vi "AlazarGetBoardKind.vi"(0 "Handle":u64, 1 "error in (no error)":errorcluster) -> (2 "Handle":u64, 3 "Board Kind":u32, 4 "Return Code":u32, 5 "error out":errorcluster)   [LabVIEW 2009]
doc: "Get a board model identifier of the board associated with a board handle."
uses:
  ATSApi.dll
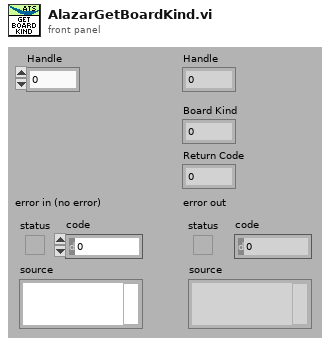
[diagram p1: front panel]
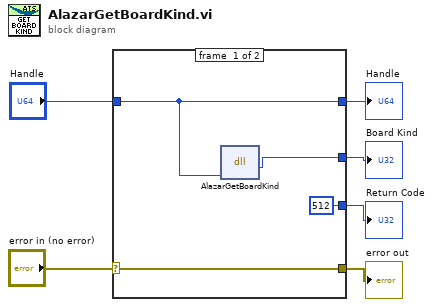
[diagram p0: block diagram]
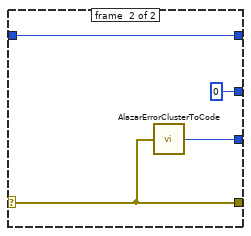
[diagram p2: hidden frame]
diagram:
  n1 = case shown="No Error" "error in (no error)" {
    selector: "error in (no error)" -> [w9 w14]
    tunnel: [w9 w14] -> w5
    tunnel: [512 w13] -> w4
    tunnel: "Handle" -> [w8 w12]
    tunnel: [w8 w12] -> w2
    tunnel: [w7 0] -> w1
    frame #0 {
      n2 = dll-call lib="ATSApi.dll" fn="AlazarGetBoardKind"("handle"=w8) -> ("return type"=w7:u32)  [unwired: 4 in, 2 out]
    }
    frame #1 {
      n3 = call "AlazarErrorClusterToCode.vi"("error in (no error)"=w14) -> ("Error Code"=w13:u32)
    }
  }
  "Handle" <- w2
  "error out" <- w5
  "Return Code" <- w4
  "Board Kind" <- w1
